vi "Write Parameters from List.vi"(8 "error in (no error)":errorcluster, 10 "Parameters from List":T1[](array[typedef]), 11 "Scan SBlock in":refnum<class "Scan SBlock.lvclass">) -> (0 "error out":errorcluster, 3 "Scan SBlock out":refnum<class "Scan SBlock.lvclass">)   [LabVIEW 2020, in "Run Utilities.lvlib" / "Scan SBlock.lvclass"]
uses:
  Scan SBlock.lvclass
  Advanced Parameters - list.ctl
  Scan SBlock.lvclass/Scan SBlock.ctl
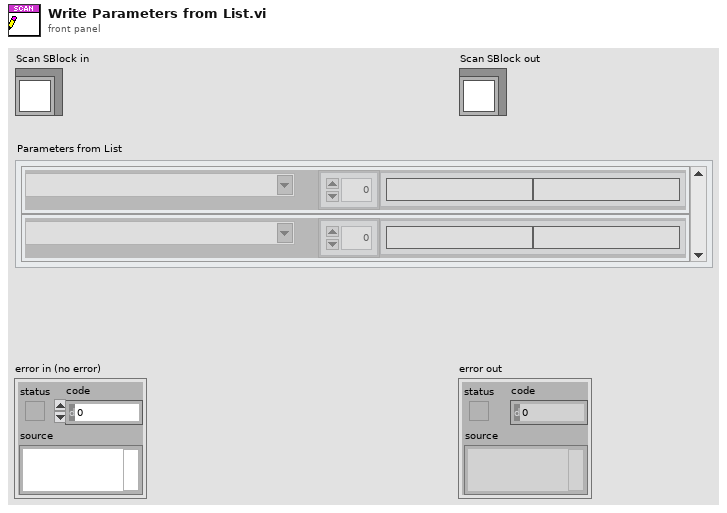
[diagram p1: front panel]
types:
  T1 = typedef "Run Utilities.lvlib/Scan SBlock.lvclass/Advanced Parameters - list.ctl" = cluster{"Param":string, "List of values":string[]}
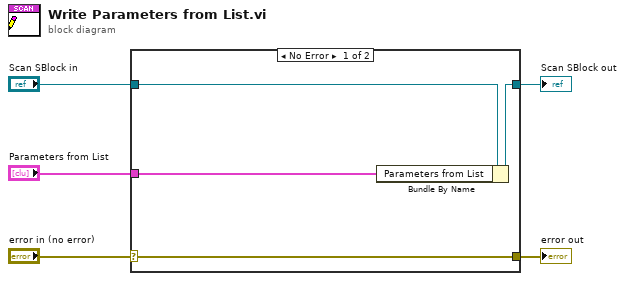
[diagram p0: block diagram]
diagram:
  n1 = case shown="No Error" "error in (no error)" {
    selector: "error in (no error)" -> [w9 w10]
    tunnel: [w9 w10] -> w4
    tunnel: [w7 w11] -> w2
    tunnel: "Scan SBlock in" -> [w8 w11]
    tunnel: "Parameters from List" -> [w6 _]
    frame No Error {
      n2 = Bundle By Name(cluster=w8, "Parameters from List"=w6) -> (w7:refnum<class "Scan SBlock.lvclass">)
    }
    frame Error {
    }
  }
  "error out" <- w4
  "Scan SBlock out" <- w2
